vi "ackExitCommand.vi"(8 "error in (no error)":errorcluster, 10 "ackcmd_Ctl":T1, 11 "SALCommunicatorController in":refnum<class "SALCommunicatorController.lvclass">) -> (0 "error out":errorcluster, 2 "function return":i32, 3 "SALCommunicatorController out":refnum<class "SALCommunicatorController.lvclass">)   [LabVIEW 2016, in "SALCommunicatorController.lvclass"]
uses:
  SALCommunicatorController.lvclass
  ts_sallv_exa/DataTypes/ackcmd.ctl
  ts_sallv_exa/SALLV_EXA.lvlib
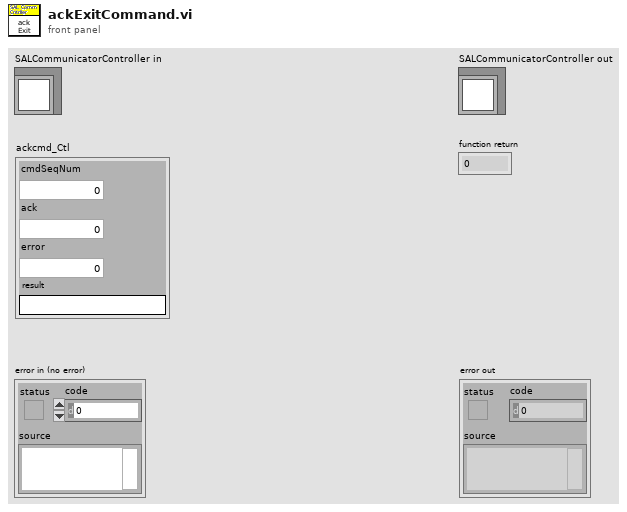
[diagram p1: front panel]
types:
  T1 = typedef "SALLV_EXA.lvlib/ackcmd.ctl" = cluster{"cmdSeqNum":i32, "ack":i32, "error":i32, "result":string}
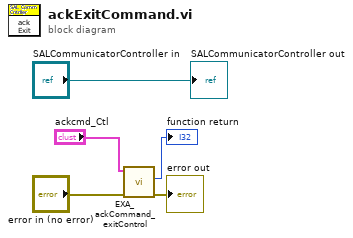
[diagram p0: block diagram]
diagram:
  n1 = call "EXA_ackCommand_exitControl.vi"("error in (no error)"="error in (no error)", "ackcmd_Ctl"="ackcmd_Ctl") -> ("error out"=→"error out":errorcluster, "function return"=→"function return":i32)  [unwired: 7 in, 1 out]
  "SALCommunicatorController out" <- "SALCommunicatorController in"
